vi "Find Enemy.vi"(7 "Primary Direction":T1, 10 "View":i32[](array[numeric]), 11 "Team Index":i32) -> (2 "Direction":T1, 3 "Found":bool)   [LabVIEW 2017, in "AntFarm_MB.lvclass"]
doc: "Reports whether an enemy is in the vicinity and some information about that enemy."
uses:
  AntFarm_MB.lvclass
  Type Defs/Direction Enum.ctl
  Type Defs/SB Type Defs.lvlib
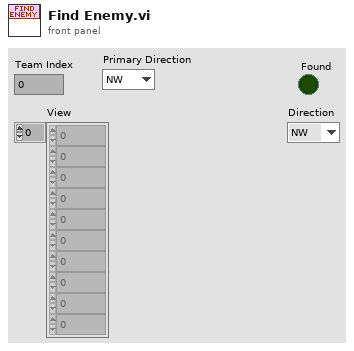
[diagram p1: front panel]
types:
  T1 = typedef "SB Type Defs.lvlib/Direction Enum.ctl" = enum16{"NW", "N", "NE", "E", "SE", "S", "SW", "W"}
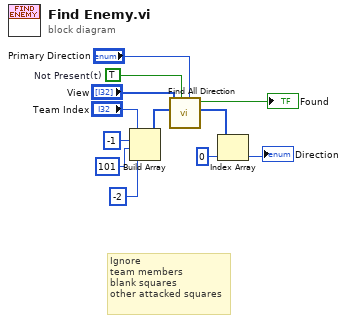
[diagram p0: block diagram]
diagram:
  w11 = TRUE  # Not Present(t)
  # "Ignore \nteam members\nblank squares\nother attacked squares"
  n1 = Build Array("Team Index", -1 ("element"), 101 ("element"), -2 ("element")) -> (w8:i32[])
  n2 = call "Find All Direction.vi"("Primary Direction"="Primary Direction", "Present(f) Not Present(t)"=w11, "Target Array"=w8, "View"="View") -> ("Direction Array Out"=w5:T1[], "Found"=→"Found":bool)  [unwired: 6 in]
  n3 = Index Array(array=w5, index=0) -> (element=→"Direction":T1)
